vi "Read Persistent Unified Actor.vi"(11 "Base Attributes in":refnum<class "Base Attributes.lvclass">) -> (2 "Persistent Unified Actor":refnum<class "Actor.lvclass">)   [LabVIEW 2025, in "jettl.lvlib" / "Base Attributes.lvlib" / "Base Attributes.lvclass"]
uses:
  Base Attributes.lvclass
  Base Attributes.lvclass/Base Attributes.ctl
  Actor/Actor.lvclass
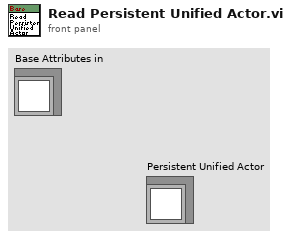
[diagram p1: front panel]
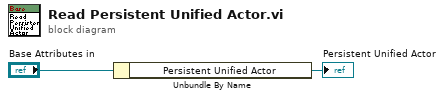
[diagram p0: block diagram]
diagram:
  n1 = Unbundle By Name("Base Attributes in") -> ("Persistent Unified Actor"=→"Persistent Unified Actor":refnum<class "Actor.lvclass">)
